vi "Change Color.vi"(0 "Control References":refnum<vi>[](array[refnum]), 1 "Temperatures":dbl[](array[numeric]), 2 "Slave ID":dbl) -> ()   [LabVIEW 2017, in "GUI.lvlib"]
uses:
  GUI.lvlib
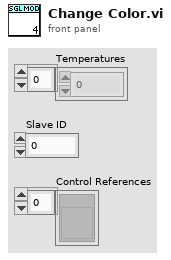
[diagram p1: front panel]
types:
  T1 = cluster{"TxA":cluster{"T1A":dbl, "T2A":dbl, "T3A":dbl, "T4A":dbl, "T5A":dbl, "T6A":dbl, "T7A":dbl, "T8A":dbl, "T9A":dbl, "T10A":dbl}, "TxO":cluster{"T1O":dbl, "T2O":dbl, "T3O":dbl, "T4O":dbl, "T5O":dbl, "T6O":dbl, "T7O":dbl, "T8O":dbl, "T9O":dbl, "T10O":dbl}}
  T2 = cluster{"T1A":dbl, "T2A":dbl, "T3A":dbl, "T4A":dbl, "T5A":dbl, "T6A":dbl, "T7A":dbl, "T8A":dbl, "T9A":dbl, "T10A":dbl}
  T3 = cluster{"T1O":dbl, "T2O":dbl, "T3O":dbl, "T4O":dbl, "T5O":dbl, "T6O":dbl, "T7O":dbl, "T8O":dbl, "T9O":dbl, "T10O":dbl}
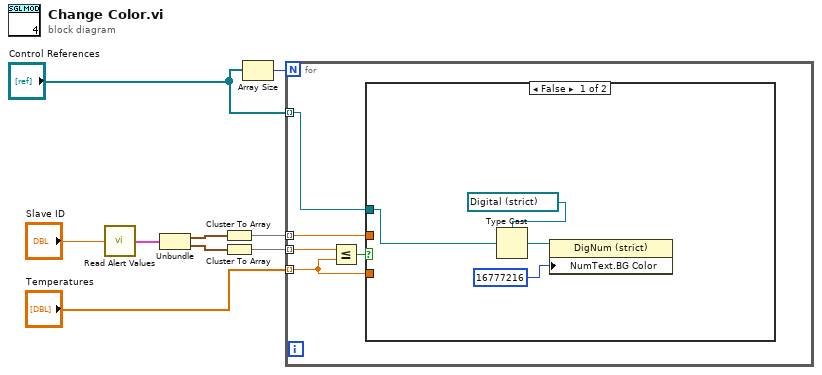
[diagram p0: block diagram]
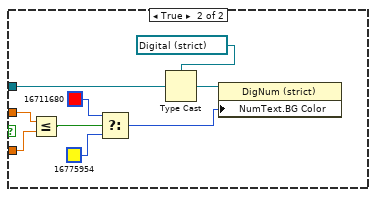
[diagram p2: hidden frame]
diagram:
  n1 = call "Read Alert Values.vi"("Section"="Slave ID") -> ("Temp Warning Values"=w4:T1)
  n2 = Unbundle(w4) -> ("TxA"=w6:T2, "TxO"=w8:T3)
  n3 = Cluster To Array(cluster=w6) -> (array=w7:dbl[])
  n4 = Cluster To Array(cluster=w8) -> (array=w9:dbl[])
  n5 = Array Size(array="Control References") -> (size(s)=w2:i32)
  n6 = for {
    N: w2 -> [_]
    tunnel: "Control References" -> [w13] mode=indexing
    tunnel: "Temperatures" -> [w11] mode=indexing
    tunnel: w7 -> [w14] mode=indexing
    tunnel: w9 -> [w10] mode=indexing
    n7 = Less Or Equal?(x=w10, y=w11) -> (x <= y?=w12:bool)
    n8 = case shown="False" w12 {
      tunnel: w11 -> [_ w20]
      tunnel: w14 -> [_ w21]
      tunnel: w13 -> [w15 w22]
      frame False {
        n9 = Type Cast(type=refnum<vi> refnum ("reference"), x=w15) -> (*(type *) &x=w18:refnum<vi>)
        n10 = property on="Property Node" class="DigNum (strict)"(reference=w18, "NumText.BG Color"=u32 16777216) -> ()  [unwired: 1 in, 2 out]
      }
      frame True {
        n11 = Less Or Equal?(x=w21, y=w20) -> (x <= y?=w19:bool)
        n12 = Select(t=u32 16711680, s=w19, f=u32 16775954) -> (s? t:f=w23:u32)
        n13 = Type Cast(type=refnum<vi> refnum ("reference"), x=w22) -> (*(type *) &x=w25:refnum<vi>)
        n14 = property on="Property Node" class="DigNum (strict)"(reference=w25, "NumText.BG Color"=w23) -> ()  [unwired: 1 in, 2 out]
      }
    }
  }
